vi "Acquire Semaphore.vi"(4 "error in (no error)":errorcluster, 5 "ms timeout (-1)":i32=-1, 7 "semaphore":T1) -> (0 "error out":errorcluster, 1 "timed out":bool, 3 "semaphore out":T1)   [LabVIEW 2020]
doc: "Acquires access to a semaphore."
uses:
  Semaphore Refnum Core.ctl
panel:
  in  "Disposed while waiting error":string="The semaphore was disposed before a lock became  available in <b>Acquire Semaphore</b>."
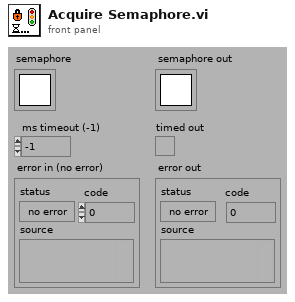
[diagram p1: front panel]
types:
  T1 = typedef "Semaphore RefNum" = refnum<k1>
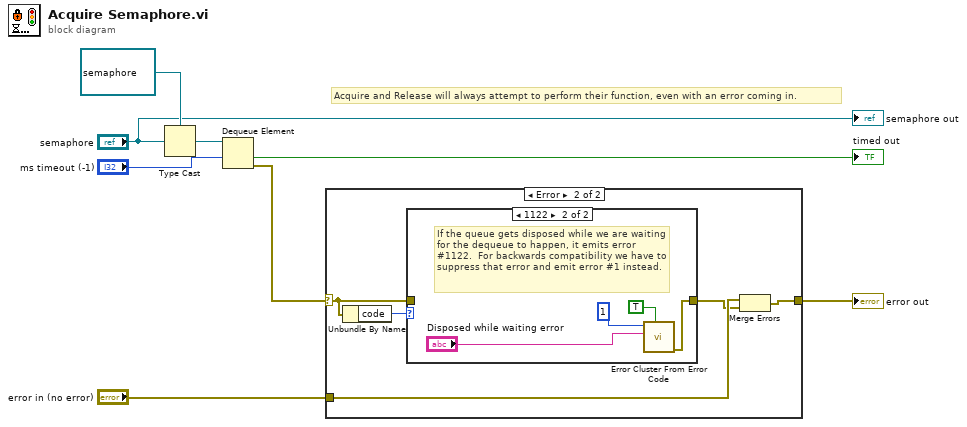
[diagram p0: block diagram]
diagram:
  w8 = refnum<queue> refnum items=["Semaphore Core"] ("queue out")
  # "Acquire and Release will always attempt to perform their function, even with an error coming in."
  n1 = Type Cast(type=w8, x="semaphore") -> (*(type *) &x=w7:refnum<queue>)
  n2 = Dequeue Element(queue=w7, timeout in ms (-1)="ms timeout (-1)") -> (timed out?=→"timed out":bool, error out=w4:errorcluster)  [unwired: 1 in, 2 out]
  n3 = case shown="Error" w4 {
    selector: w4 -> [_ w13]
    tunnel: [w9 w10] -> w2
    tunnel: "error in (no error)" -> [w9 w12]
    frame No Error {
      # "If we have no errors, propagate the value"
    }
    frame Error {
      n4 = Unbundle By Name(w13) -> ("code"=w14:i32)
      n5 = case shown="1122" w14 {
        tunnel: w13 -> [w15 _]
        tunnel: [w15 w19] -> w11
        frame 0, Default {
          # "let other errors go without modification"
        }
        frame 1122 {
          # "If the queue gets disposed while we are waiting for the dequeue to happen, it emits error #1122.  For backwards compatibility we have to suppress that error and emit error #1 instead."
          n6 = call "Error Cluster From Error Code.vi"("show call chain? (False)"=TRUE, "error message (\"\")"="Disposed while waiting error", "error code (0)"=1) -> ("error out"=w19:errorcluster)  [unwired: 1 in, 5 out]
        }
      }
      n7 = Merge Errors(w12, w11) -> (w10:errorcluster)
    }
  }
  "error out" <- w2
  "semaphore out" <- "semaphore"
